vi "CSM - Global Log Event.vi"(8 "Error in":errorcluster caption="Error in (no error)") -> (0 "Error out":errorcluster, 3 "JKISM Global Log Event":refnum<user-event>)   [LabVIEW 2014, in "Communicable State Machine.lvlib"]
doc: "Obtain CSM Global Log Event Reference.\n\n<b>Inputs:</b>\n - <b>Error in</b>: Error cluster\n\n<b>Outputs:</b>\n - <b>CSM Global Log Event</b>: User event reference for CSM global log.\n - <b>Error out</b>: Error cluster"
uses:
  Communicable State Machine.lvlib
  _Support/Typedef/_CSM_GlobalLog_MSG.ctl
  _Support/Typedef/_CSM_GlobalLog_MSG_TYPE.ctl
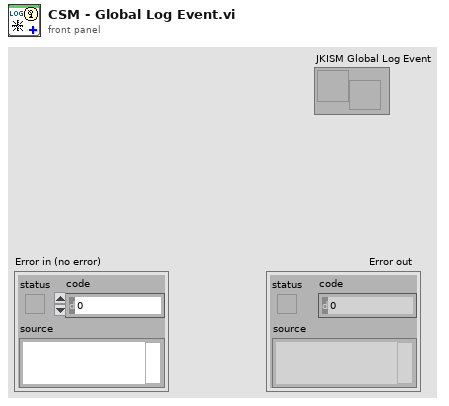
[diagram p1: front panel]
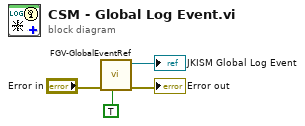
[diagram p0: block diagram]
diagram:
  n1 = call "FGV-GlobalEventRef.vi"("Create(F)"=TRUE, "error in (no error)"="Error in") -> ("error out"=→"Error out":errorcluster, "JKISM Global Log Event"=→"JKISM Global Log Event":refnum<user-event>)  [unwired: 8 in]
